vi "Catch Object.vi"(11 "error in (no error)":errorcluster) -> (4 "LVx Command":refnum<class "LVx.lvclass">, 15 "error out":errorcluster)   [LabVIEW 2011, in "LVx.lvlib" / "LVx.lvclass"]
uses:
  LVx.lvclass
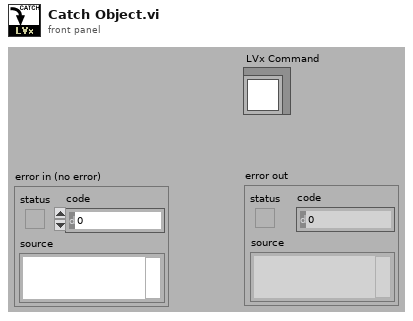
[diagram p1: front panel]
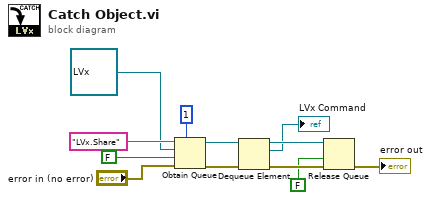
[diagram p0: block diagram]
diagram:
  n1 = Obtain Queue(max queue size (-1, unlimited)=1, name (unnamed)="LVx.Share", element data type=refnum<class "LVx.lvclass"> refnum ("LVx.lvlib:LVx.lvclass"), create if not found? (T)=FALSE, error in (no error)="error in (no error)") -> (queue out=w8:refnum<queue>, error out=w7:errorcluster)  [unwired: 1 out]
  n2 = Dequeue Element(queue=w8, error in (no error)=w7) -> (queue out=w6:refnum<queue>, element=→"LVx Command":refnum<class "LVx.lvclass">, error out=w5:errorcluster)  [unwired: 2 out]
  n3 = Release Queue(queue=w6, force destroy? (F)=FALSE, error in (no error)=w5) -> (error out=→"error out":errorcluster)  [unwired: 2 out]
